vi "Format String Insert Into 3 (SubVI).vi"(4 "NIM":string, 5 "Boolean":bool, 6 "Nama":string, 7 "Foto":path, 8 "error in (no error)":errorcluster, 9 "Alamat":string, 10 "Email":string, 11 "Refnum in":T1) -> (0 "error out":errorcluster, 2 "resulting string":string, 3 "Refnum out":T1)   [LabVIEW 2024]
uses:
  <vilib>/addons/database/Connection.llb/Conn ObjectReference.ctl
  <vilib>/addons/database/Connection.llb/Conn Execute.vi
  <vilib>/addons/database/NI_Database_API.lvlib
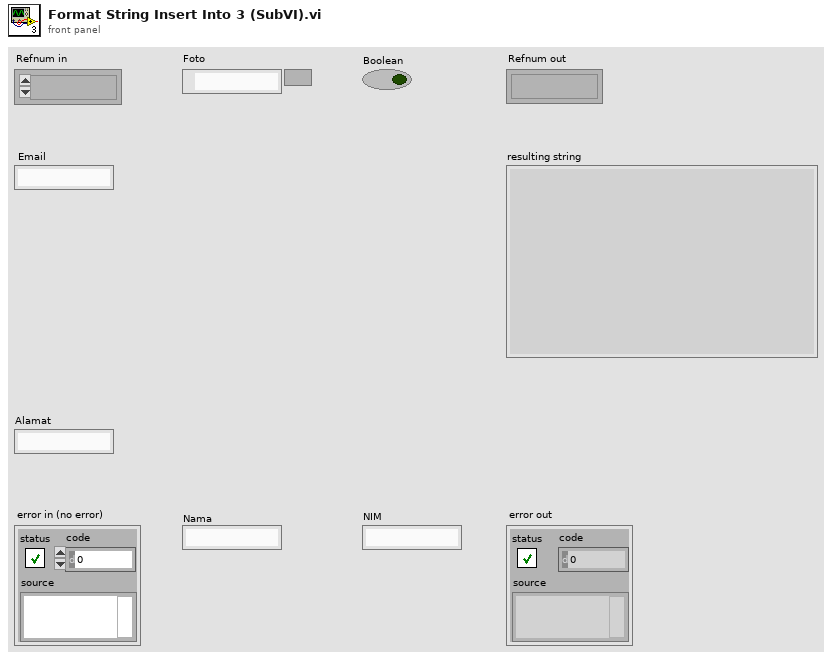
[diagram p1: front panel]
types:
  T1 = typedef "NI_Database_API.lvlib/Conn ObjectReference.ctl" = refnum<k1>
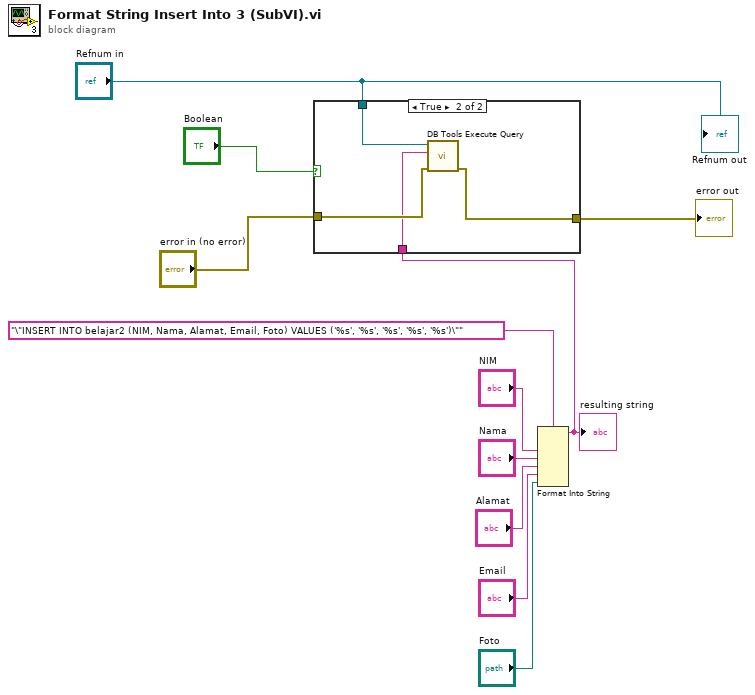
[diagram p0: block diagram]
diagram:
  n1 = Format Into String(format string="\"INSERT INTO belajar2 (NIM, Nama, Alamat, Email, Foto) VALUES ('%s', '%s', '%s', '%s', '%s')\"", "NIM", "Nama", "Alamat", "Email", "Foto") -> (resulting string=w11:string)  [unwired: 2 in, 1 out]
  "resulting string" <- w11
  n2 = case shown="True" "Boolean" {
    tunnel: "Refnum in" -> [_ w16]
    tunnel: "error in (no error)" -> [w12 w15]
    tunnel: [w12 w14] -> w3
    tunnel: w11 -> [_ w13]
    frame False {
    }
    frame True {
      n3 = call-poly <vilib>:"DB Tools Execute Query.vi"("error in (no error)"=w15, "SQL query"=w13, "connection reference"=w16) -> ("error out"=w14:errorcluster)  [unwired: 5 in, 1 out]
    }
  }
  "error out" <- w3
  "Refnum out" <- "Refnum in"
